vi "Clear Scalar Channels.vi"(8 "error in":errorcluster, 11 "FPGA Addon refnum in":T1=18446744073709551615 format="%.0x") -> (0 "error out":errorcluster, 3 "FPGA Addon refnum out":T1=18446744073709551615 format="%.0x")   [LabVIEW 2018, in "Scripting API.lvlib"]
uses:
  Scripting API.lvlib
  <vilib>/NI Veristand/Custom Device API/Custom Device Item Ref.ctl
  Addon/Addon Shared/SubVIs/Constants.vi
  <vilib>/NI/NI VeriStand Advanced SysDef API/_SubVIs/SysDef.Search.GUID.vi
  Addon/Addon Shared/FPGA Addon Shared.lvlib
  <vilib>/NI/NI VeriStand Advanced SysDef API/SysDef API/Advanced System Definition.lvlib
  <vilib>/NI Veristand/Custom Device API/Custom Device API.lvlib
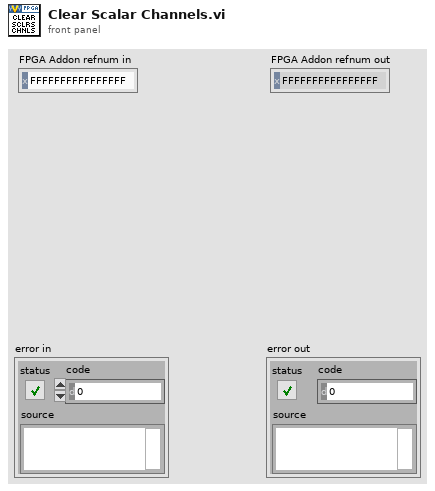
[diagram p1: front panel]
types:
  T1 = typedef "Custom Device API.lvlib/Custom Device Item Ref.ctl" = u64
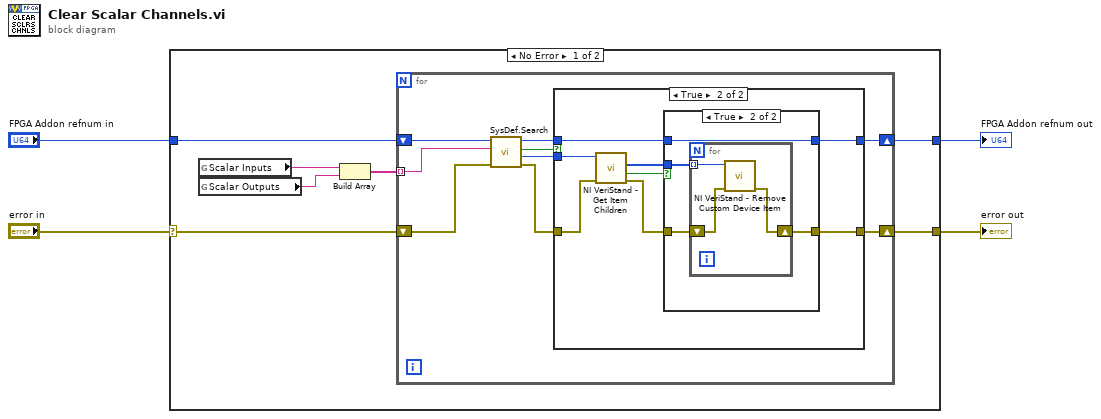
[diagram p0: block diagram]
diagram:
  n1 = case shown="No Error" "error in" {
    selector: "error in" -> [w7 w40]
    tunnel: "FPGA Addon refnum in" -> [w9 w41]
    tunnel: [w6 w41] -> w2
    tunnel: [w5 w40] -> w1
    frame No Error {
      n2 = global read "Constants.vi" "Scalar Inputs"() -> (w11:string)
      n3 = global read "Constants.vi" "Scalar Outputs"() -> (w10:string)
      n4 = Build Array(w11, w10) -> (w8:string[])
      n5 = for {
        tunnel: w8 -> [w20] mode=indexing
        shift-right: [w14] -> w6
        shift-left: w9 -> [w19]
        shift-right: [w12] -> w5
        shift-left: w7 -> [w17]
        n6 = call-poly <vilib>:"SysDef.Search.vi"("error in (no error)"=w17, "GUID"=w20, "nodeID"=w19) -> ("error out"=w16:errorcluster, "Value out"=w18:u64, "nodeID out"=w15:u64, "Found?"=w13:bool)  [unwired: 5 in]
        n7 = case shown="True" w13 {
          tunnel: w18 -> [_ w30]
          tunnel: w16 -> [w21 w28]
          tunnel: w15 -> [w22 w25]
          tunnel: [w22 w24] -> w14
          tunnel: [w21 w23] -> w12
          frame False {
          }
          frame True {
            n8 = call <vilib>:"NI VeriStand - Get Item Children.vi"("error in (no error)"=w28, "Item Ref in"=w30) -> ("error out"=w27:errorcluster, "Child Refs"=w29:T1[], "Found"=w26:bool)  [unwired: 6 in, 1 out]
            n9 = case shown="True" w26 {
              tunnel: w29 -> [_ w36]
              tunnel: w27 -> [w31 w35]
              tunnel: w25 -> [w32 w34]
              tunnel: [w32 w34] -> w24
              tunnel: [w31 w33] -> w23
              frame False {
              }
              frame True {
                n10 = for {
                  tunnel: w36 -> [w39] mode=indexing
                  shift-right: [w37] -> w33
                  shift-left: w35 -> [w38]
                  n11 = call <vilib>:"NI VeriStand - Remove Custom Device Item.vi"("error in (no error)"=w38, "Item Ref in"=w39) -> ("error out"=w37:errorcluster)  [unwired: 8 in, 1 out]
                }
              }
            }
          }
        }
      }
    }
    frame Error {
    }
  }
  "error out" <- w1
  "FPGA Addon refnum out" <- w2
